vi "EventLogger-Write.vi"(7 "Device reference":refnum<vi>, 8 "error in (no error)":errorcluster, 9 "Eventstring":string) -> (0 "error out":errorcluster)   [LabVIEW 2015]
doc: "Generates a timestamp pulse and writes an eventstring."
uses:
  Typedefs/EventLogger.ctl
  Rack/Typedefs/OutputRequest refnum.ctl
  Rack/Typedefs/OutputRequest.ctl
  Rack/Typedefs/InputData cluster.ctl
  Rack/Methods/Port drivers/DigitalInput-DataCluster.ctl
panel:
  # "Timestamp"
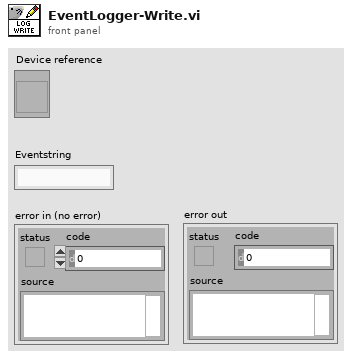
[diagram p1: front panel]
types:
  T1 = typedef "EventLogger.ctl" = cluster{"Settings":cluster{"Portname":string, "Index":i32}, "OutputRequest event ref":T2, "InputData reference":refnum<vi>}
  T2 = typedef "OutputRequest refnum.ctl" = refnum<user-event>
  T3 = typedef "OutputRequest.ctl" = cluster{"Target":string, "Command":string}
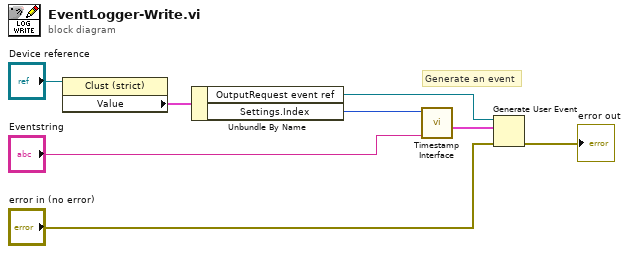
[diagram p0: block diagram]
diagram:
  # "Generate an event"
  n1 = property class="Clust (strict)"(reference="Device reference") -> ("Value"=w7:T1)  [unwired: 1 in, 2 out]
  n2 = Unbundle By Name(w7) -> ("OutputRequest event ref"=w3:T2, "Settings.Index"=w6:i32)
  n3 = call "Timestamp Interface.vi"("Eventstring"="Eventstring", "Port index"=w6) -> ("OutputRequest"=w4:T3)  [unwired: 9 in]
  n4 = Generate User Event(user event=w3, event data cluster=w4, error in="error in (no error)") -> (error out=→"error out":errorcluster)  [unwired: 1 in, 1 out]
